vi "Read VI Refnum.vi"(8 "error in (no error)":errorcluster, 11 "BD_PAPAS_USD_ES in":refnum<class "BD_PAPAS_USD_ES.lvclass">) -> (0 "error out":errorcluster, 2 "VI Refnum":refnum<vi>, 3 "BD_PAPAS_USD_ES out":refnum<class "BD_PAPAS_USD_ES.lvclass">)   [LabVIEW 2019, in "BD_PAPAS_USD_ES.lvlib" / "BD_PAPAS_USD_ES.lvclass"]
uses:
  BD_PAPAS_USD_ES.lvclass
  BD_PAPAS_USD_ES.lvclass/BD_PAPAS_USD_ES.ctl
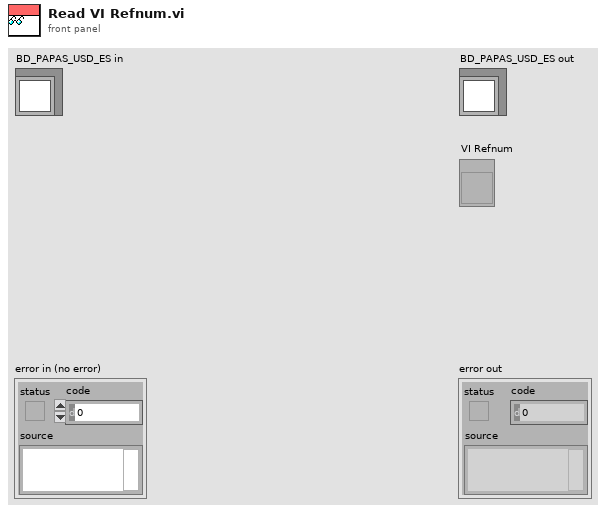
[diagram p1: front panel]
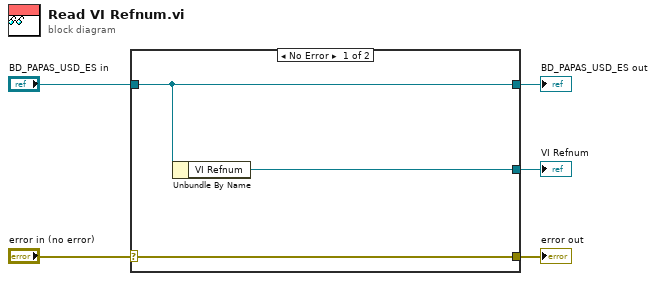
[diagram p0: block diagram]
diagram:
  n1 = case shown="No Error" "error in (no error)" {
    selector: "error in (no error)" -> [w8 w9]
    tunnel: [w8 w9] -> w4
    tunnel: [w7 w10] -> w2
    tunnel: "BD_PAPAS_USD_ES in" -> [w7 w10]
    tunnel: [w6 _] -> w1
    frame No Error {
      n2 = Unbundle By Name(w7) -> ("VI Refnum"=w6:refnum<vi>)
    }
    frame Error {
    }
  }
  "error out" <- w4
  "BD_PAPAS_USD_ES out" <- w2
  "VI Refnum" <- w1
